vi "SwerveDriveRotate.vi"(0 "Strafe Joystick Axes":cluster{"X":dbl, "Y":dbl}, 1 "Center of Rotation Joystick Axes":cluster{"X":dbl, "Y":dbl}, 2 "Trigger Axes":cluster{"Left":dbl, "Right":dbl}, 4 "Angle (degrees; 0 = right)":dbl, 5 "error in (no error)":errorcluster, 6 "Strafe Multiplier":dbl, 7 "FieldCentric? (T)":bool=TRUE, 8 "Rotation Multiplier":dbl, 9 "Steering Motor Refs":T1[](array[typedef]), 10 "Max Wheel Speed":dbl, 11 "Speed Motor Refs":T1[](array[typedef])) -> (14 "Steering Motor Setpoints":dbl[](array[numeric]), 15 "Speed Motor Setpoints":dbl[](array[numeric]), 16 "Speed Chart":cluster{dbl, "Encoder Velocity":dbl}[](graph), 17 "Position Chart":cluster{dbl, "Encoder Velocity":dbl}[](graph), 19 "error out":errorcluster)   [LabVIEW 2016, in "Team900SwerveDrive.lvlib"]
uses:
  Team900SwerveDrive.lvlib
  <vilib>/Rock Robotics/WPI/MotorControl/WPI_MotorControlDeviceRef.ctl
  <vilib>/Rock Robotics/WPI/MotorControl/WPI_MotorControlType.ctl
  <vilib>/Rock Robotics/SystemInterfaces/DIO/FPGA_DIOPWMChannel.ctl
  <vilib>/Rock Robotics/WPI/PWM/WPI_PWMDeadband.ctl
  <vilib>/Rock Robotics/WPI/ThirdParty/CanMotor/TalonSRX/WPI_CANTalonSRX_APIControlMode.ctl
  <vilib>/Rock Robotics/Network Tables/NT Write Numeric Array.vi
  Logitech/F510/F510-X.vi
  OnButton/OnButtonSingle.vi
panel:
  in  "Speed PID":cluster{"P":dbl, "I":dbl, "D":dbl}={"P"=0.0275, "I"=0.000115, "D"=0.682955}
  in  "Speed PID 2":cluster{"P":dbl, "I":dbl, "D":dbl}={"P"=0.0275, "I"=0.000115, "D"=0.682955}
  in  "% VBus":dbl
  # "Most basic version of SwerveDrive, expects two joystick inputs, one for\nstrafe, one for the center of rotation (can be left unwired if you just\nwant the robot to rotate around its center), and triggers for rotation\n(pressing the right trigger rotates clockwise, left trigger counterclockwise)\n\nIf the FieldCentric control is false, then up on the joystick is forward for the\nrobot; if it is true then the strafe vector is rotated based on the Angle input\nso that up on the strafe joystick drives in a constant direction regardless\nof robot heading."
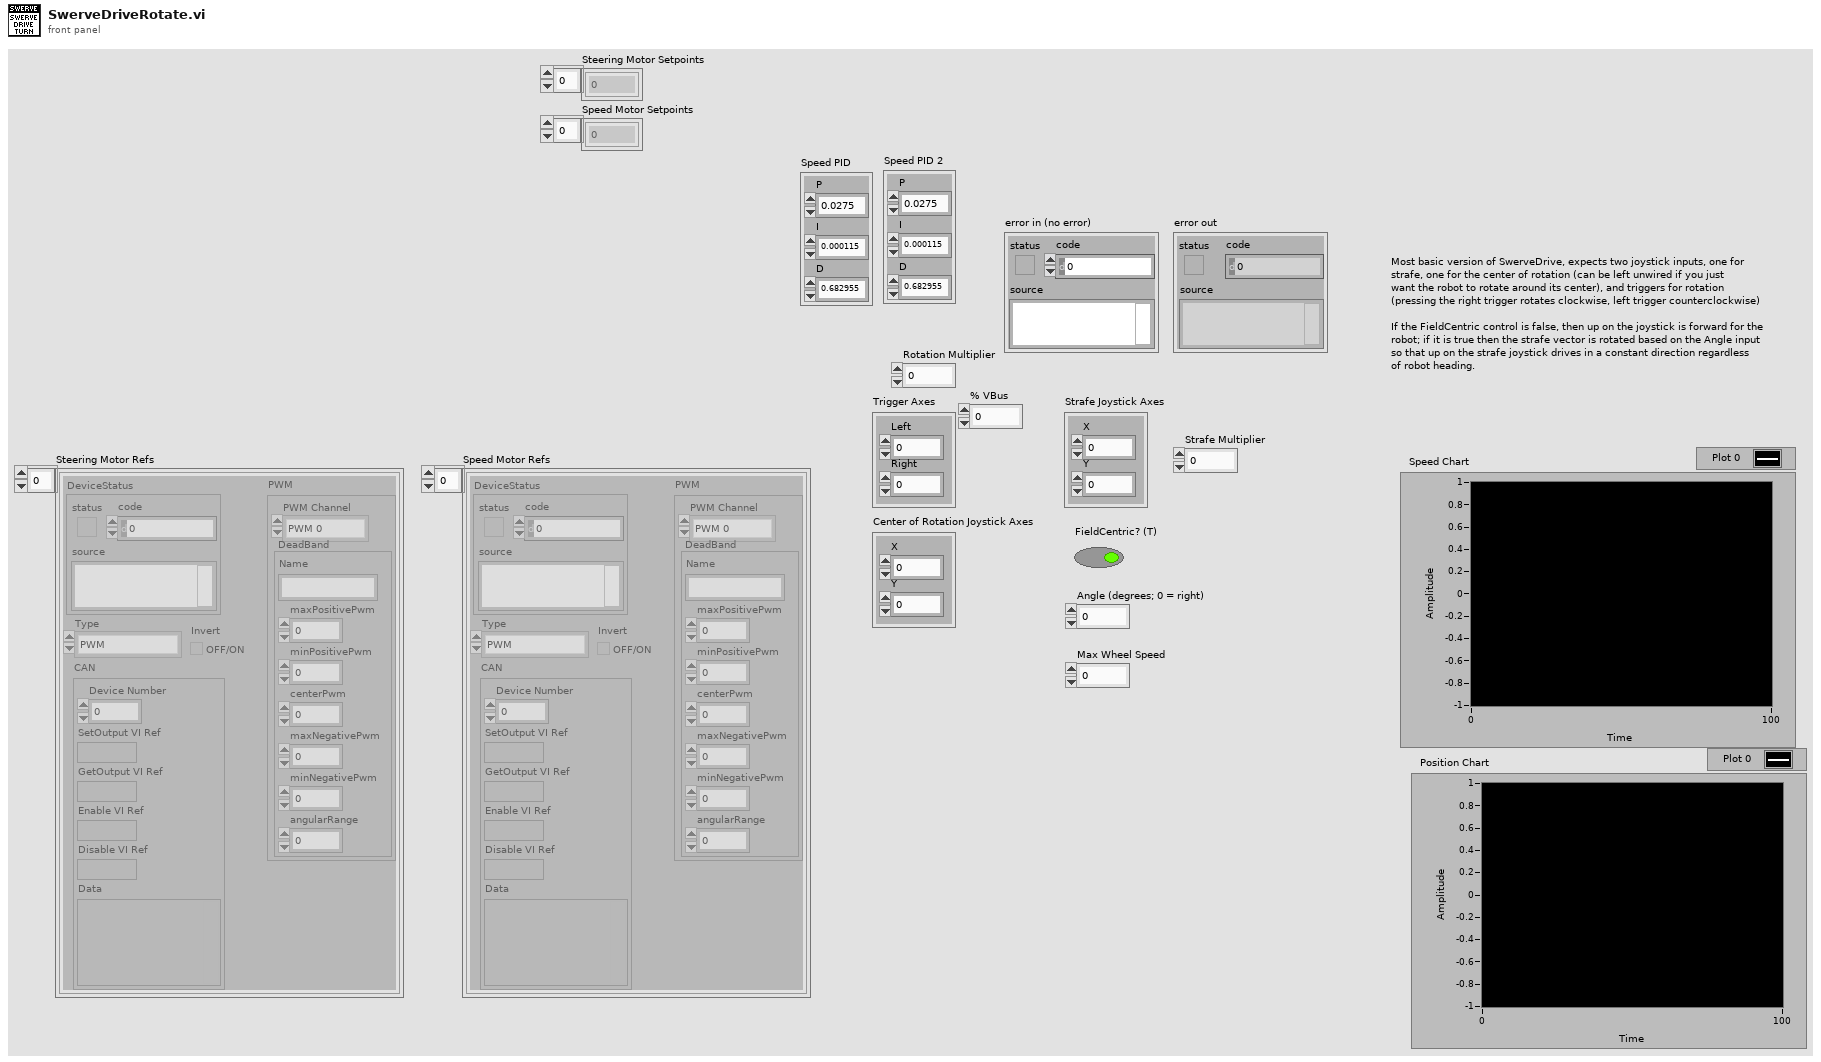
[diagram p1: front panel]
types:
  T1 = typedef "WPI_MotorControlDeviceRef.ctl" = cluster{"DeviceStatus":errorcluster, "Type":T2, "PWM":cluster{"PWM Channel":T3, "DeadBand":T4}, "CAN":cluster{"Device Number":u8, "SetOutput VI Ref":variant, "GetOutput VI Ref":variant, "Enable VI Ref":variant, "Disable VI Ref":variant, "Data":variant}, "Invert":bool}
  T2 = typedef "WPI_MotorControlType.ctl" = enum16{"PWM", "CAN"}
  T3 = typedef "FPGA_DIOPWMChannel.ctl" = enum8{"PWM 0", "PWM 1", "PWM 2", "PWM 3", "PWM 4", "PWM 5", "PWM 6", "PWM 7", "PWM 8", "PWM 9", "PWM MXP 0", "PWM MXP 1", "PWM MXP 2", "PWM MXP 3", "PWM MXP 4", "PWM MXP 5", "PWM MXP 6", "PWM MXP 7", "PWM MXP 8", "PWM MXP 9", "Invalid"}
  T4 = typedef "WPI_PWMDeadband.ctl" = cluster{"Name":string, "maxPositivePwm":i32, "minPositivePwm":i32, "centerPwm":i32, "maxNegativePwm":i32, "minNegativePwm":i32, "angularRange":u16}
  T5 = cluster{"Up":bool, "Right":bool, "Down":bool, "Left":bool}
  T6 = cluster{"FL Steering":T1, "FR Steering":T1, "RL Steering":T1, "RR Steering":T1}
  T7 = cluster{"FL Speed":T1, "FR Speed":T1, "RL Speed":T1, "RR Speed":T1}
  T8 = cluster{"Speed Motor Refs[0]":T1, "Speed Motor Refs[1]":T1, "Speed Motor Refs[2]":T1, "Speed Motor Refs[3]":T1}
  T9 = cluster{"Steering Motor Refs[0]":T1, "Steering Motor Refs[1]":T1, "Steering Motor Refs[2]":T1, "Steering Motor Refs[3]":T1}
  T10 = typedef "WPI_CANTalonSRX_GlobalStatus.ctl" = cluster{"Applied Throttle":dbl, "Module Enabled":bool, "CAN Error":errorcluster, "Closed Loop Error":dbl, "Forward Limit Switch Closed":bool, "Reverse Limit Switch Closed":bool, "Sensor Position":dbl, "Sensor Velocity":dbl, "Current":dbl, "Sticky Fault - Over Temp":bool, "Sticky Fault - Under Voltage":bool, "Sticky Fault - Forward Limit":bool, "Sticky Fault - Reverse Limit":bool, "Sticky Fault - Forward Soft Limit":bool, "Sticky Fault - Reverse Soft Limit":bool, "Brake is Enabled":bool, "Encoder Position":dbl, "Encoder Velocity":dbl, "Encoder Index Count":dbl, "Encoder A Pin State":bool, "Encoder B Pin State":bool, "Encoder Index Pin State":bool, "Analog In":dbl, "Analog In Velocity":dbl, "Temperature (C)":dbl, "Battery Voltage":dbl, "Control 5 Is Supported":bool, "Current Profile Slot Select":dbl, "Pos Div 8":bool, "Vel Div 4":bool, "Pulse Width Position":i32, "Pulse Width Velocity":i32, "Pulse Width Rise To Rise (us)":i32, "Pulse Width Rise To Fall (us)":i32, "Mot Prof Active Is Under Run":bool, "Mot Prof Active Has Under Run":bool, "Mot Prof Active Is Last":bool, "Mot Prof Active Velocity Only":bool, "Mot Prof Active Is Valid":bool, "Mot Prof Buffer Is Full":bool, "Mot Prof Active Profile Slot Select":i32, "Mot Prof NextID":i32, "Mot Prof Count":i32, "Mot Prof Active Velocity":dbl, "Mot Prof Active Position":dbl, "Mot Prof Output Enable":i32}
  T11 = cluster{"output angle":dbl, "Encoder Velocity":dbl}
  T12 = typedef "WPI_CANTalonSRX_APIControlMode.ctl" = enum8{"Percent VBus", "Speed", "Position", "Slave", "Unchanged / Invalid", "Voltage Compensation", "Current", "Motion Profile"}
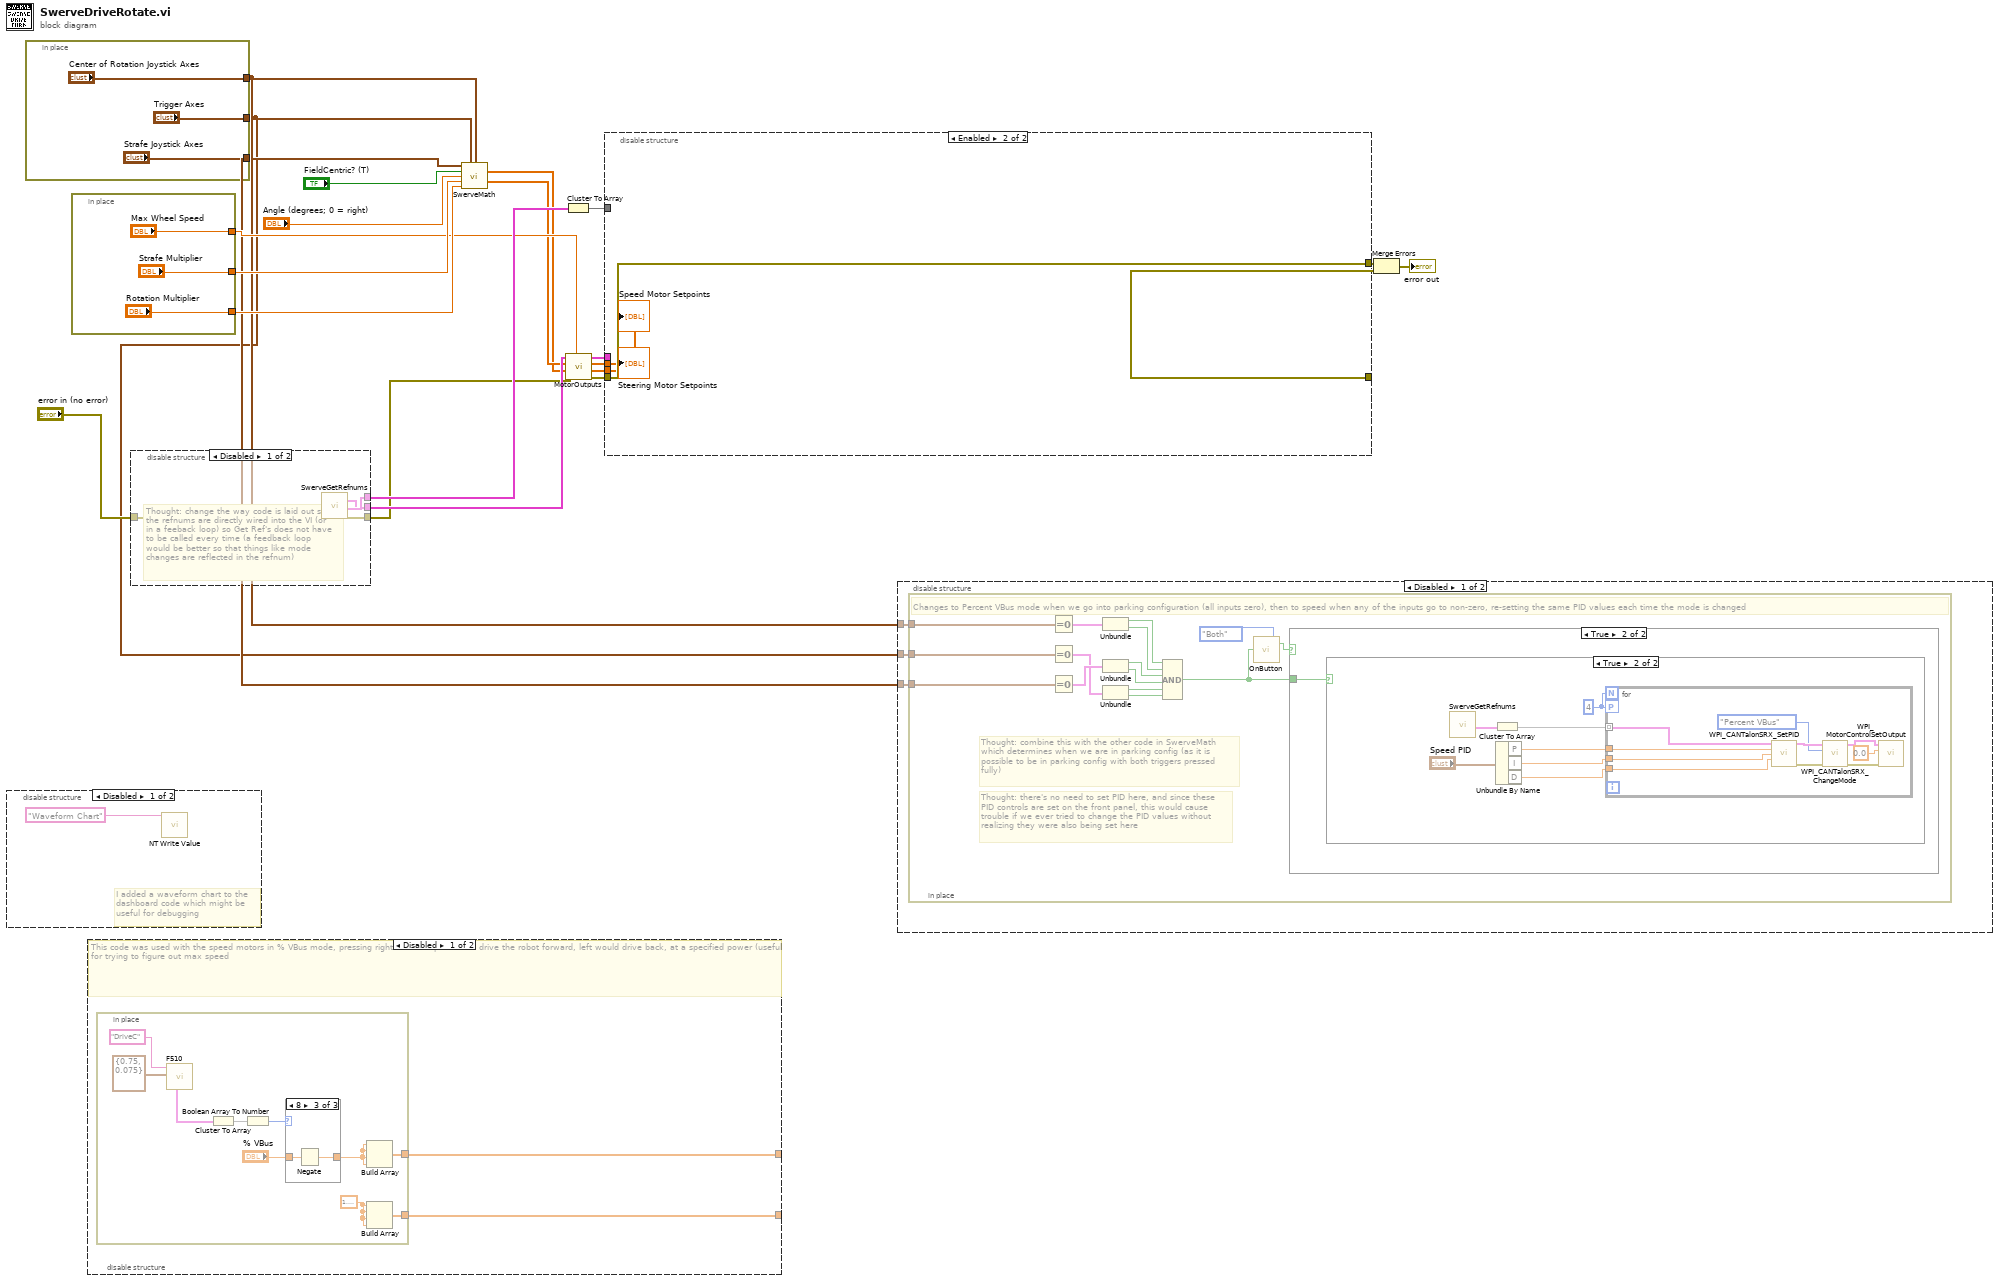
[diagram p0: block diagram]
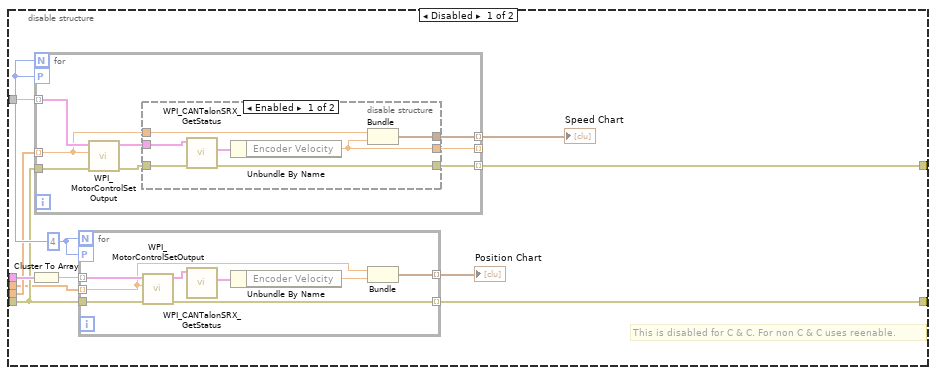
[diagram p2: hidden frame]
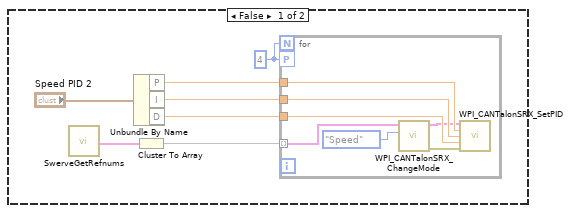
[diagram p5: hidden frame]
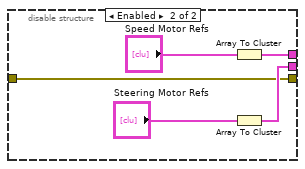
[diagram p7: hidden frame]
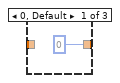
[diagram p9: hidden frame]
diagram:
  n1 = disable-structure shown="Disabled" {
    frame Disabled {
      # "I added a waveform chart to the\ndashboard code which might be\nuseful for debugging"
      n2 = call-poly <vilib>:"NT Write Value.vi"("Name"="Waveform Chart") -> ()  [unwired: 10 in, 1 out]
    }
    frame Enabled {
    }
  }
  n3 = in-place {
    in-place-border: ["Center of Rotation Joystick Axes"] -> w3
    in-place-border: ["Strafe Joystick Axes"] -> w2
    in-place-border: ["Trigger Axes"] -> w1
  }
  n4 = in-place {
    in-place-border: ["Max Wheel Speed"] -> w8
    in-place-border: ["Rotation Multiplier"] -> w15
    in-place-border: ["Strafe Multiplier"] -> w14
  }
  n5 = disable-structure shown="Disabled" {
    disable-tunnel: [w31 _] -> _
    disable-tunnel: [w30 _] -> _
    frame Disabled {
      # "This code was used with the speed motors in % VBus mode, pressing right on the D-pad would drive the robot forward, left would drive back, at a specified power (useful for trying to figure out max speed"
      n6 = in-place {
        in-place-border: [w39] -> w31
        in-place-border: [w37] -> w30
        w38 = 1.5707963267948966
        n7 = call-poly "F510.vi"("Deadzone Scale Cluster"=cluster{"Scale":dbl, "Deadzone":dbl} {"Scale"=0.75, "Deadzone"=0.075}, "refnum name"="DriveC") -> ("D-Pad Buttons"=w35:T5)  [unwired: 3 in, 6 out]
        n8 = Cluster To Array(cluster=w35) -> (array=w36:bool[])
        n9 = Boolean Array To Number(Boolean array=w36) -> (number=w34:u32)
        n10 = case shown="8" w34 {
          tunnel: "% VBus" -> [_ w43 w45]
          tunnel: [0 w43 w44] -> w33
          frame 0, Default {
          }
          frame 2 {
          }
          frame 8 {
            n11 = Negate(x=w45) -> (-x=w44:dbl)
          }
        }
        n12 = Build Array(w33, w33, w33, w33) -> (w39:dbl[])
        n13 = Build Array(w38, w38, w38, w38) -> (w37:dbl[])
      }
    }
    frame Enabled {
    }
  }
  n14 = disable-structure shown="Disabled" {
    disable-tunnel: [w49 w51] -> w19
    disable-tunnel: "error in (no error)" -> [w48 w50]
    disable-tunnel: [w47 w53] -> w13
    disable-tunnel: [w46 w50] -> w11
    frame Disabled {
      # "Thought: change the way code is laid out so\nthe refnums are directly wired into the VI (or\nin a feeback loop) so Get Ref's does not have\nto be called every time (a feedback loop\nwould be better so that things like mode \nchanges are reflected in the refnum)"
      n15 = call "SwerveGetRefnums.vi"("error in (no error)"=w48) -> ("Steering"=w47:T6, "Speed"=w49:T7, "error out"=w46:errorcluster)  [unwired: 8 in, 8 out]
    }
    frame Enabled {
      n16 = Array To Cluster(array="Speed Motor Refs") -> (cluster=w51:T8)
      n17 = Array To Cluster(array="Steering Motor Refs") -> (cluster=w53:T9)
    }
  }
  n18 = call "SwerveMath.vi"("Strafe Joystick Axes"=w2, "Trigger Axes"=w1, "Center of Rotation Joystick"=w3, "FieldCentric? (T)"="FieldCentric? (T)", "Angle (degrees; 0 = right)"="Angle (degrees; 0 = right)", "Strafe Multiplier"=w14, "Rotation Multiplier"=w15) -> ("Motor Speeds"=w5:dbl[], "Motor Angles"=w6:dbl[])  [unwired: 7 in]
  n19 = Cluster To Array(cluster=w19) -> (array=w17:T1[])
  n20 = call "MotorOutputs.vi"("Max Wheel Speed"=w8, "error in (no error)"=w11, "Motor Speeds"=w5, "Target Angles"=w6, "Steering Refnums In"=w13) -> ("error out"=w10:errorcluster, "Speed Motor Setpoints"=w9:dbl[], "Steering Motor Setpoints"=w4:dbl[], "Steering Refnums Out"=w12:T6)  [unwired: 3 in]
  n21 = disable-structure shown="Enabled" {
    disable-tunnel: [w65 w92] -> w18
    disable-tunnel: w17 -> [w64 _]
    disable-tunnel: w12 -> [w62 _]
    disable-tunnel: w10 -> [w60 w92]
    disable-tunnel: w9 -> [w59 w90]
    disable-tunnel: [w58 _] -> w7
    disable-tunnel: w4 -> [w57 w91]
    frame Disabled {
      w63 = 4
      # "This is disabled for C & C. For non C & C uses reenable."
      n22 = Cluster To Array(cluster=w62) -> (array=w61:T1[])
      n23 = for {
        N: w63 -> [_]
        tunnel: w60 -> [w81]
        tunnel: [w78] -> w65 mode=indexing
        workers-P: w63 -> [_]
        tunnel: w64 -> [w80] mode=indexing
        tunnel: [w76] -> _ mode=indexing
        tunnel: [w75] -> w56 mode=indexing
        tunnel: w59 -> [w74] mode=indexing
        n24 = call <vilib>:"WPI_MotorControlSetOutput.vi"("error in (no error)"=w81, "Output"=w74, "MotorControlDevRef"=w80) -> ("error out"=w79:errorcluster, "MotorControlDevRef"=w77:T1)  [unwired: 6 in, 1 out]
        n25 = disable-structure shown="Enabled" {
          disable-tunnel: w79 -> [w88 w89]
          disable-tunnel: [w87 w89] -> w78
          disable-tunnel: w77 -> [w86 _]
          disable-tunnel: [w84 _] -> w76
          disable-tunnel: [w82 _] -> w75
          disable-tunnel: w74 -> [w83 _]
          frame Enabled {
            n26 = call <vilib>:"WPI_CANTalonSRX_GetStatus.vi"("error in (no error)"=w88, "CAN Talon SRX Ref"=w86) -> ("error out"=w87:errorcluster, "Talon SRX Status"=w85:T10)  [unwired: 7 in, 1 out]
            n27 = Unbundle By Name(w85) -> ("Encoder Velocity"=w84:dbl)
            n28 = Bundle(w83, "Encoder Velocity"=w84) -> (w82:cluster{dbl, "Encoder Velocity":dbl})  [unwired: 1 in]
          }
          frame Disabled {
          }
        }
      }
      "Speed Chart" <- w56
      n29 = for {
        N: w63 -> [_]
        tunnel: w60 -> [w73]
        workers-P: w63 -> [_]
        tunnel: w61 -> [w72] mode=indexing
        tunnel: w57 -> [w67] mode=indexing
        tunnel: [w71] -> w58 mode=indexing
        tunnel: [w66] -> w55 mode=indexing
        n30 = call <vilib>:"WPI_MotorControlSetOutput.vi"("error in (no error)"=w73, "Output"=w67, "MotorControlDevRef"=w72) -> ("error out"=w71:errorcluster, "MotorControlDevRef"=w69:T1)  [unwired: 6 in, 1 out]
        n31 = call <vilib>:"WPI_CANTalonSRX_GetStatus.vi"("CAN Talon SRX Ref"=w69) -> ("Talon SRX Status"=w70:T10)  [unwired: 8 in, 2 out]
        n32 = Unbundle By Name(w70) -> ("Encoder Velocity"=w68:dbl)
        n33 = Bundle("output angle"=w67, "Encoder Velocity"=w68) -> (w66:T11)  [unwired: 1 in]
      }
      "Position Chart" <- w55
    }
    frame Enabled {
      "Steering Motor Setpoints" <- w91
      "Speed Motor Setpoints" <- w90
    }
  }
  n34 = disable-structure shown="Disabled" {
    disable-tunnel: w3 -> [w95 _]
    disable-tunnel: w2 -> [w94 _]
    disable-tunnel: w1 -> [w93 _]
    frame Disabled {
      n35 = in-place {
        in-place-border: w95 -> [w98]
        in-place-border: w94 -> [w97]
        in-place-border: w93 -> [w96]
        # "Thought: there's no need to set PID here, and since these\nPID controls are set on the front panel, this would cause\ntrouble if we ever tried to change the PID values without\nrealizing they were also being set here"
        # "Thought: combine this with the other code in SwerveMath\nwhich determines when we are in parking config (as it is\npossible to be in parking config with both triggers pressed\nfully)"
        # "Changes to Percent VBus mode when we go into parking configuration (all inputs zero), then to speed when any of the inputs go to non-zero, re-setting the same PID values each time the mode is changed"
        n36 = Equal To 0?(x=w98) -> (x = 0?=w102:cluster{"X":bool, "Y":bool})
        n37 = Equal To 0?(x=w96) -> (x = 0?=w100:cluster{"Left":bool, "Right":bool})
        n38 = Equal To 0?(x=w97) -> (x = 0?=w101:cluster{"X":bool, "Y":bool})
        n39 = Unbundle(w102) -> ("X"=w106:bool, "Y"=w105:bool)
        n40 = Unbundle(w101) -> ("X"=w108:bool, "Y"=w107:bool)
        n41 = Unbundle(w100) -> ("Left"=w104:bool, "Right"=w103:bool)
        n42 = Compound Arithmetic op=AND(w106, w105, w108, w107, w104, w103) -> (w99:bool)
        n43 = call-poly "OnButton.vi"("Input"=w99, "Released"=enum16{"Press", "Release", "Both"}."Both" ("Mode")) -> ("Pressed"=w110:bool)
        n44 = case shown="True" w110 {
          tunnel: w99 -> [_ w111]
          frame False {
          }
          frame True {
            n45 = case shown="True" w111 {
              frame False {
                w112 = 4
                n46 = call "SwerveGetRefnums.vi"() -> ("Speed"=w117:T7)  [unwired: 9 in, 10 out]
                n47 = Unbundle By Name("Speed PID 2") -> ("P"=w116:dbl, "I"=w115:dbl, "D"=w114:dbl)
                n48 = Cluster To Array(cluster=w117) -> (array=w118:T1[])
                n49 = for {
                  N: w112 -> [_]
                  workers-P: w112 -> [_]
                  tunnel: w118 -> [w121] mode=indexing
                  tunnel: w116 -> [w123]
                  tunnel: w115 -> [w124]
                  tunnel: w114 -> [w125]
                  n50 = call <vilib>:"WPI_CANTalonSRX_ChangeMode.vi"("Control Mode"=WPI_CANTalonSRX_APIControlMode."Speed", "CAN Talon SRX Ref"=w121) -> ("error out"=w119:errorcluster, "CAN Talon SRX Ref"=w120:T1)  [unwired: 8 in]
                  n51 = call <vilib>:"WPI_CANTalonSRX_SetPID.vi"("CAN Talon SRX Ref"=w120, "P"=w123, "I"=w124, "D"=w125, "error in (no error)"=w119) -> ()  [unwired: 9 in, 2 out]
                }
              }
              frame True {
                w126 = 4
                n52 = call "SwerveGetRefnums.vi"() -> ("Speed"=w131:T7)  [unwired: 9 in, 10 out]
                n53 = Cluster To Array(cluster=w131) -> (array=w132:T1[])
                n54 = Unbundle By Name("Speed PID") -> ("P"=w130:dbl, "I"=w129:dbl, "D"=w128:dbl)
                n55 = for {
                  N: w126 -> [_]
                  workers-P: w126 -> [_]
                  tunnel: w132 -> [w142] mode=indexing
                  tunnel: w130 -> [w139]
                  tunnel: w129 -> [w140]
                  tunnel: w128 -> [w141]
                  n56 = call <vilib>:"WPI_CANTalonSRX_SetPID.vi"("CAN Talon SRX Ref"=w142, "P"=w139, "I"=w140, "D"=w141) -> ("CAN Talon SRX Ref"=w138:T1, "error out"=w137:errorcluster)  [unwired: 10 in]
                  n57 = call <vilib>:"WPI_CANTalonSRX_ChangeMode.vi"("error in (no error)"=w137, "Control Mode"=WPI_CANTalonSRX_APIControlMode."Percent VBus", "CAN Talon SRX Ref"=w138) -> ("error out"=w135:errorcluster, "CAN Talon SRX Ref"=w134:T1)  [unwired: 7 in]
                  n58 = call <vilib>:"WPI_MotorControlSetOutput.vi"("error in (no error)"=w135, "Output"=0.0, "MotorControlDevRef"=w134) -> ()  [unwired: 6 in, 3 out]
                }
              }
            }
          }
        }
      }
    }
    frame Enabled {
    }
  }
  n59 = Merge Errors(w18, w7) -> (→"error out":errorcluster)
